vi "Read Single Digital Input and Get High Time.vi"(0 "Lines":tag, 5 "Rate (Hz)":dbl=1000.0 format="%0.2f", 7 "Samples":i32=1000, 11 "Error In":errorcluster) -> (4 "High Time (s)":dbl, 15 "Error Out":errorcluster)   [LabVIEW 2016]
doc: "This VI reads a single digital input and provides an output of the high time in seconds for that line."
uses:
  <vilib>/DAQmx/read.llb/DAQmx Read (Digital Wfm 1Chan NSamp).vi
  <vilib>/DAQmx/create/channels.llb/DAQmx Create Channel (DI-Digital Input).vi
  <vilib>/DAQmx/configure/timing.llb/DAQmx Timing (Sample Clock).vi
  <vilib>/DAQmx/miscellaneous.llb/DAQmx Fill In Error Info.vi
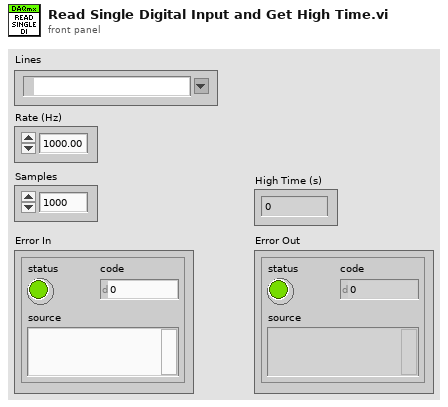
[diagram p1: front panel]
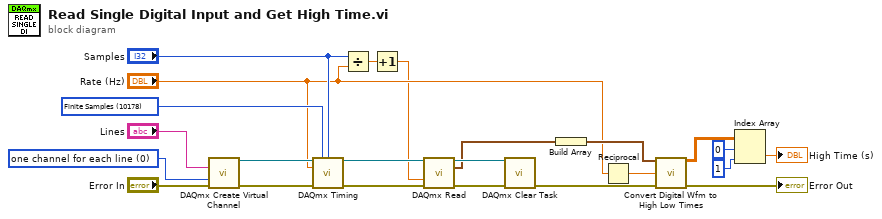
[diagram p0: block diagram]
diagram:
  w14 = 10178 items=["Finite Samples"=10178, "Continuous Samples"=10123, "Hardware Timed Single Point"=12522] ("sample mode")
  w23 = 0 items=["one channel for each line", "one channel for all lines"] ("line grouping")
  n1 = call-poly <vilib>:"DAQmx Create Virtual Channel.vi"("lines"="Lines", "line grouping"=w23, "error in"="Error In") -> ("task out"=w18:refnum<k21>, "error out"=w17:errorcluster)  [unwired: 11 in]
  n2 = call-poly <vilib>:"DAQmx Timing.vi"("task/channels in"=w18, "sample mode"=w14, "samples per channel"="Samples", "rate"="Rate (Hz)", "error in"=w17) -> ("task out"=w16:refnum<k21>, "error out"=w15:errorcluster)  [unwired: 9 in]
  n3 = Divide(x="Samples", y="Rate (Hz)") -> (x/y=w6:dbl)
  n4 = Increment(x=w6) -> (x+1=w5:dbl)
  n5 = call-poly <vilib>:"DAQmx Read.vi"("task/channels in"=w16, "timeout"=w5, "error in"=w15) -> ("task out"=w21:refnum<k21>, "data"=w13:digitalwaveform, "error out"=w22:errorcluster)  [unwired: 10 in]
  n6 = call <vilib>:"DAQmx Clear Task.vi"("task in"=w21, "error in"=w22) -> ("error out"=w10:errorcluster)  [unwired: 13 in]
  n7 = Build Array(w13) -> (w12:digitalwaveform[])
  n8 = Reciprocal(x="Rate (Hz)") -> (1/x=w11:dbl)
  n9 = call "Convert Digital Wfm to High Low Times.vi"("Digital Waveform In"=w12, "Dt"=w11, "Error In"=w10) -> ("HL Raw Output"=w4:dbl[][], "Error Out"=→"Error Out":errorcluster)  [unwired: 11 in]
  n10 = Index Array(array=w4, index (row)=0 ("disabled index (row)"), index (col)=1 ("disabled index (col)")) -> (element=→"High Time (s)":dbl)
